vi "PantherLAB_Log - Duplicate DQMH Module.vi"(4 "Original Tester":path, 6 "Original Library":path, 9 "New Tester":path, 10 "New Library":path, 11 "Project":refnum<vi>) -> (0 "error out":errorcluster)   [LabVIEW 2016]
doc: "_____\nCreated using DQMH Framework: Event Scripter 7.1.0.1450."
uses:
  PantherDashboard Scripting Hooks/PantherLAB_Log.lvlib
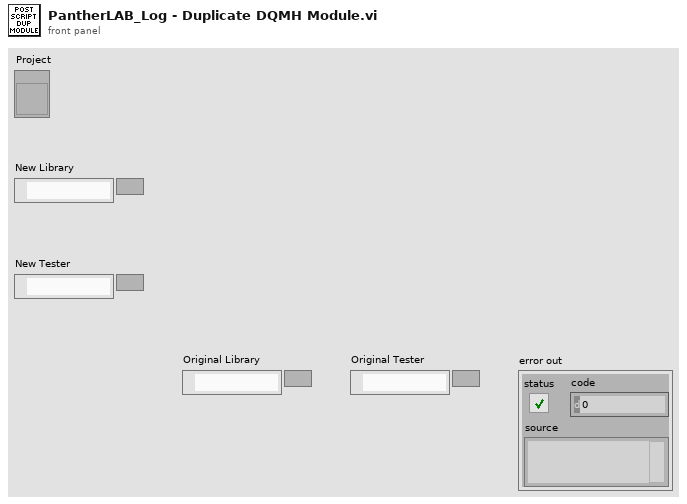
[diagram p1: front panel]
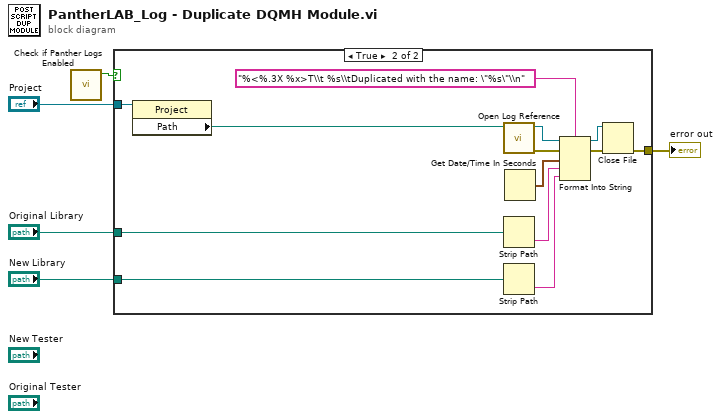
[diagram p0: block diagram]
diagram:
  n1 = call "Check if Panther Logs Enabled.vi"() -> ("PantherLogs Enabled?"=w4:bool)  [unwired: 11 in]
  n2 = case shown="True" w4 {
    tunnel: "Project" -> [_ w11]
    tunnel: "Original Library" -> [_ w9]
    tunnel: "New Library" -> [_ w6]
    tunnel: [_ w16] -> w5
    frame False {
    }
    frame True {
      n3 = property class="Project"(reference=w11) -> ("Path"=w12:path)  [unwired: 1 in, 2 out]
      n4 = call "Open Log Reference.vi"("Project Path"=w12) -> ("error out"=w18:errorcluster, "File Reference"=w15:refnum<file>)  [unwired: 9 in]
      n5 = Strip Path(path=w9) -> (name=w8:string)  [unwired: 1 out]
      n6 = Strip Path(path=w6) -> (name=w7:string)  [unwired: 1 out]
      n7 = Get Date/Time In Seconds() -> (seconds since 1Jan1904=w13:timestamp)
      n8 = Format Into String(format string="%<%.3X %x>T\\t %s\\tDuplicated with the name: \"%s\"\\n", initial string=w15, error in=w18, w13, w8, w7) -> (resulting string=w14:refnum<file>, error out=w17:errorcluster)
      n9 = Close File(refnum=w14, error in=w17) -> (error out=w16:errorcluster)  [unwired: 1 out]
    }
  }
  "error out" <- w5
